vi "Differential Current Sense.vi"(0 "Waveform Array":waveform(dbl)[](array[waveform]), 7 "Idle Offset Voltage":dbl) -> (4 "Waveform Array Out":waveform(dbl)[](array[waveform]))   [LabVIEW 2010]
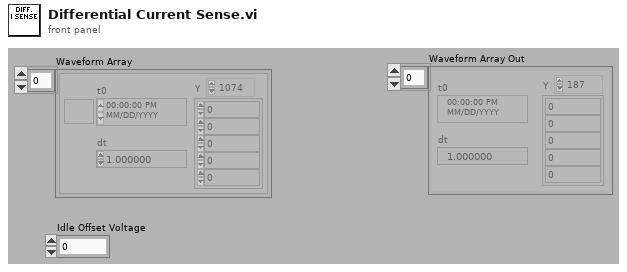
[diagram p1: front panel]
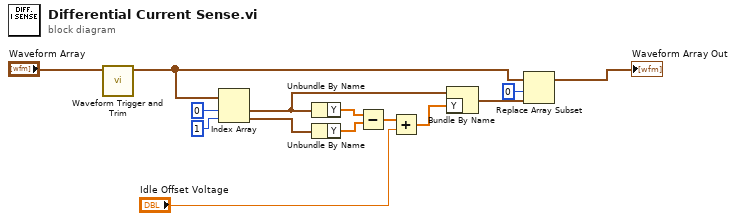
[diagram p0: block diagram]
diagram:
  n1 = call "Waveform Trigger and Trim.vi"("Waveforms In"="Waveform Array") -> ("Waveforms Out"=w1:waveform(dbl)[])  [unwired: 10 in]
  n2 = Index Array(array=w1, index #1=0 ("index"), index #2=1 ("index")) -> (element #1=w6:waveform(dbl), element #2=w12:waveform(dbl))
  n3 = Unbundle By Name(w6) -> ("Y"=w11:dbl[])
  n4 = Unbundle By Name(w12) -> ("Y"=w10:dbl[])
  n5 = Subtract(x=w11, y=w10) -> (x-y=w9:dbl[])
  n6 = Add(x=w9, y="Idle Offset Voltage") -> (x+y=w7:dbl[])
  n7 = Bundle By Name(cluster=w6, "Y"=w7) -> (w4:waveform(dbl))
  n8 = Replace Array Subset(array=w1, new element=w4, index=0) -> (→"Waveform Array Out":waveform(dbl)[])
